vi "Acquire Analyze Visualize - Your Turn Solution.vi"() -> ()   [LabVIEW 2020]
uses:
  <vilib>/DAQmx/read.llb/DAQmx Read (Analog DBL 1Chan 1Samp).vi
  <vilib>/DAQmx/miscellaneous.llb/DAQmx Fill In Error Info.vi
panel:
  out "Current Temperature (deg F)":dbl format="%#_2g"
  out "Current Temperature (deg C)":dbl format="%#_2f"
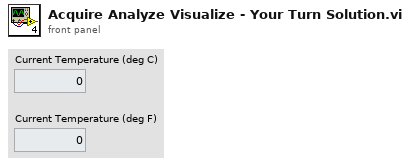
[diagram p1: front panel]
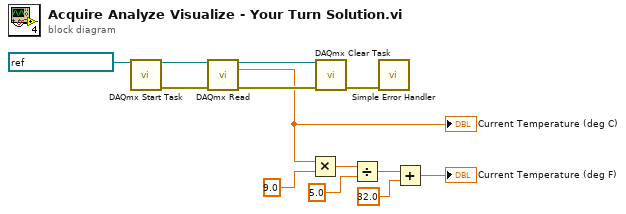
[diagram p0: block diagram]
diagram:
  n1 = call <vilib>:"DAQmx Start Task.vi"("task/channels in"=refnum<k21> "Thermocouple" ("DAQmx Task Name")) -> ("task out"=w10:refnum<k21>, "error out"=w12:errorcluster)  [unwired: 13 in]
  n2 = call-poly <vilib>:"DAQmx Read.vi"("task/channels in"=w10, "error in"=w12) -> ("task out"=w11:refnum<k21>, "data"=w8:dbl, "error out"=w13:errorcluster)  [unwired: 11 in]
  "Current Temperature (deg C)" <- w8
  n3 = Multiply(x=w8, y=9.0) -> (x*y=w6:dbl)
  n4 = call <vilib>:"DAQmx Clear Task.vi"("task in"=w11, "error in"=w13) -> ("error out"=w1:errorcluster)  [unwired: 13 in]
  n5 = Divide(x=w6, y=5.0) -> (x/y=w4:dbl)
  n6 = call <vilib>:"Simple Error Handler.vi"("error in (no error)"=w1) -> ()  [unwired: 4 in, 5 out]
  n7 = Add(x=w4, y=32.0) -> (x+y=→"Current Temperature (deg F)":dbl)
